vi "Determine Die Type by Prober Coordinate.vi"(7 "Die_Coordinates":string[](array[string]), 8 "error in (no error)":errorcluster, 10 "VISA resource name":refnum<visa-resource-name>="GPIB1::11::INSTR", 11 "USID":T1 max=15) -> (0 "error out":errorcluster, 3 "Package_Type":string)   [LabVIEW 2013]
uses:
  Controls/USID.ctl
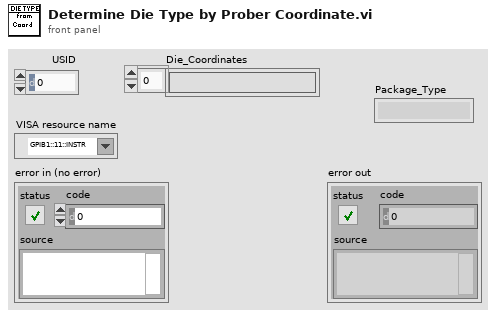
[diagram p1: front panel]
types:
  T1 = typedef "USID.ctl" = u8
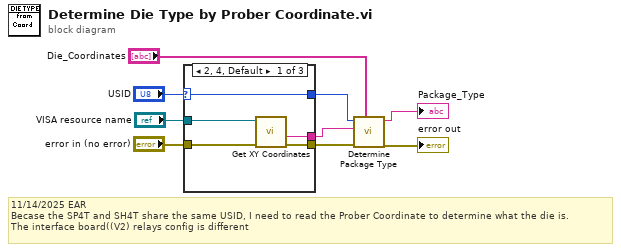
[diagram p0: block diagram]
diagram:
  # "11/14/2025 EAR\nBecase the SP4T and SH4T share the same USID, I need to read the Prober Coordinate to determine what the die is.\nThe interface board((V2) relays config is different"
  n1 = case shown="2, 4, Default" "USID" {
    selector: "USID" -> [w12 w16 w18]
    tunnel: [w14 w15 w17] -> w8
    tunnel: [w13 _ _] -> w6
    tunnel: [w12 w16 w18] -> w7
    tunnel: "error in (no error)" -> [w11 w15 w17]
    tunnel: "VISA resource name" -> [w10 _ _]
    frame 2, 4, Default {
      n2 = call "Get XY Coordinates.vi"("error in (no error)"=w11, "VISA resource name"=w10) -> ("error out"=w14:errorcluster, "X_Y"=w13:string)  [unwired: 6 in, 2 out]
    }
    frame 7, 9 {
    }
    frame 1, 14 {
    }
  }
  n3 = call "Determine Package Type.vi"("Die_Coordinates"="Die_Coordinates", "error in (no error)"=w8, "Die_X_Y"=w6, "USID"=w7) -> ("error out"=→"error out":errorcluster, "Package_Type"=→"Package_Type":string)  [unwired: 6 in]
